vi "2-Rotina de processamento dos dados de caracterização.vi"() -> ()   [LabVIEW 2011]
uses:
  <vilib>/Analysis/NI_AALBase.lvlib
  <vilib>/Analysis/baseanly.llb/Mean (DBL).vi
  <vilib>/Analysis/Matrix/Datatypes/RealMatrix.ctl
  <vilib>/Analysis/Matrix/NI_Matrix.lvlib
  <vilib>/Analysis/NI_AALPro.lvlib
  <vilib>/Analysis/polynomials.llb/1D Polynomial Evaluation (DBL).vi
panel:
  in  "Quantidade \nde Ciclos":dbl
  in  "Massas-padrão\nutilizadas (kg)":dbl[](array[numeric])
  out "Mensagem":string
  out "Regressão Linear:":string
  out "Coeficiente de Determinação:":dbl
  out "Tensão e \nForça do Sinal":cluster{"Y":dbl[], "Y":dbl[]}[](graph)
  # "*1"
  # "*x"
  # "*(x^2)"
  # "*(x^3)"
  # "ROTINA DE PROCESSAMENTO DOS DADOS DE CARACTERIZAÇÃO"
  # "(Um ciclo\ncorresponde\na um \ncarreganento\nseguido de um \ndescarregamento)"
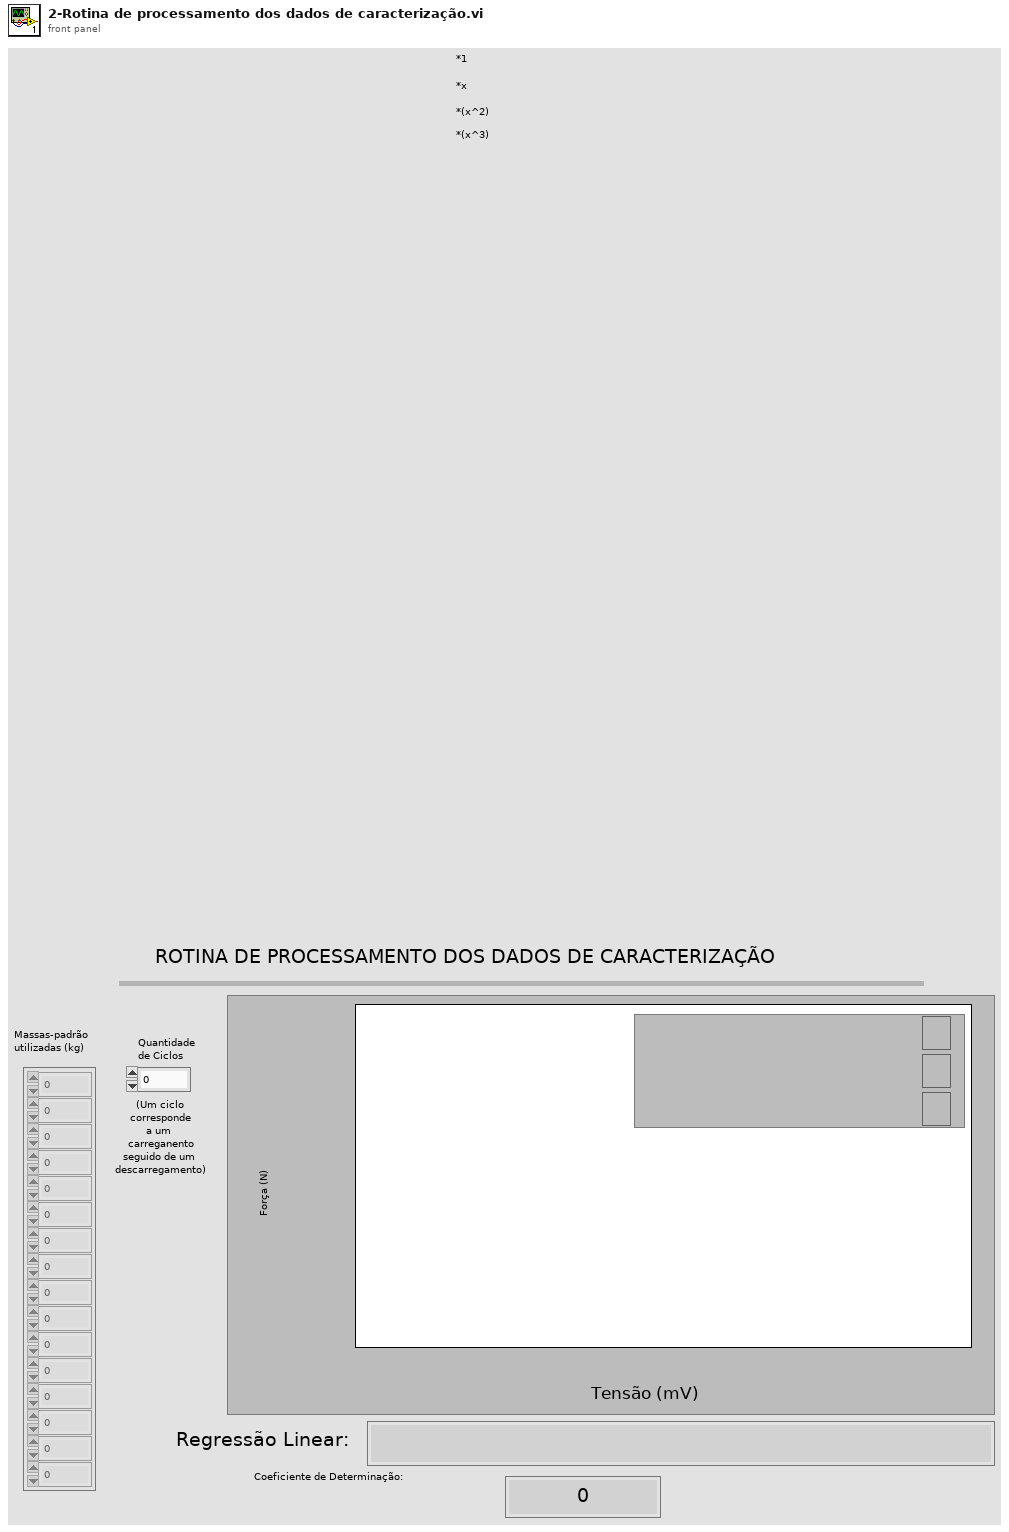
[diagram p1: front panel]
types:
  T1 = typedef "NI_Matrix.lvlib/RealMatrix.ctl" = dbl[][]
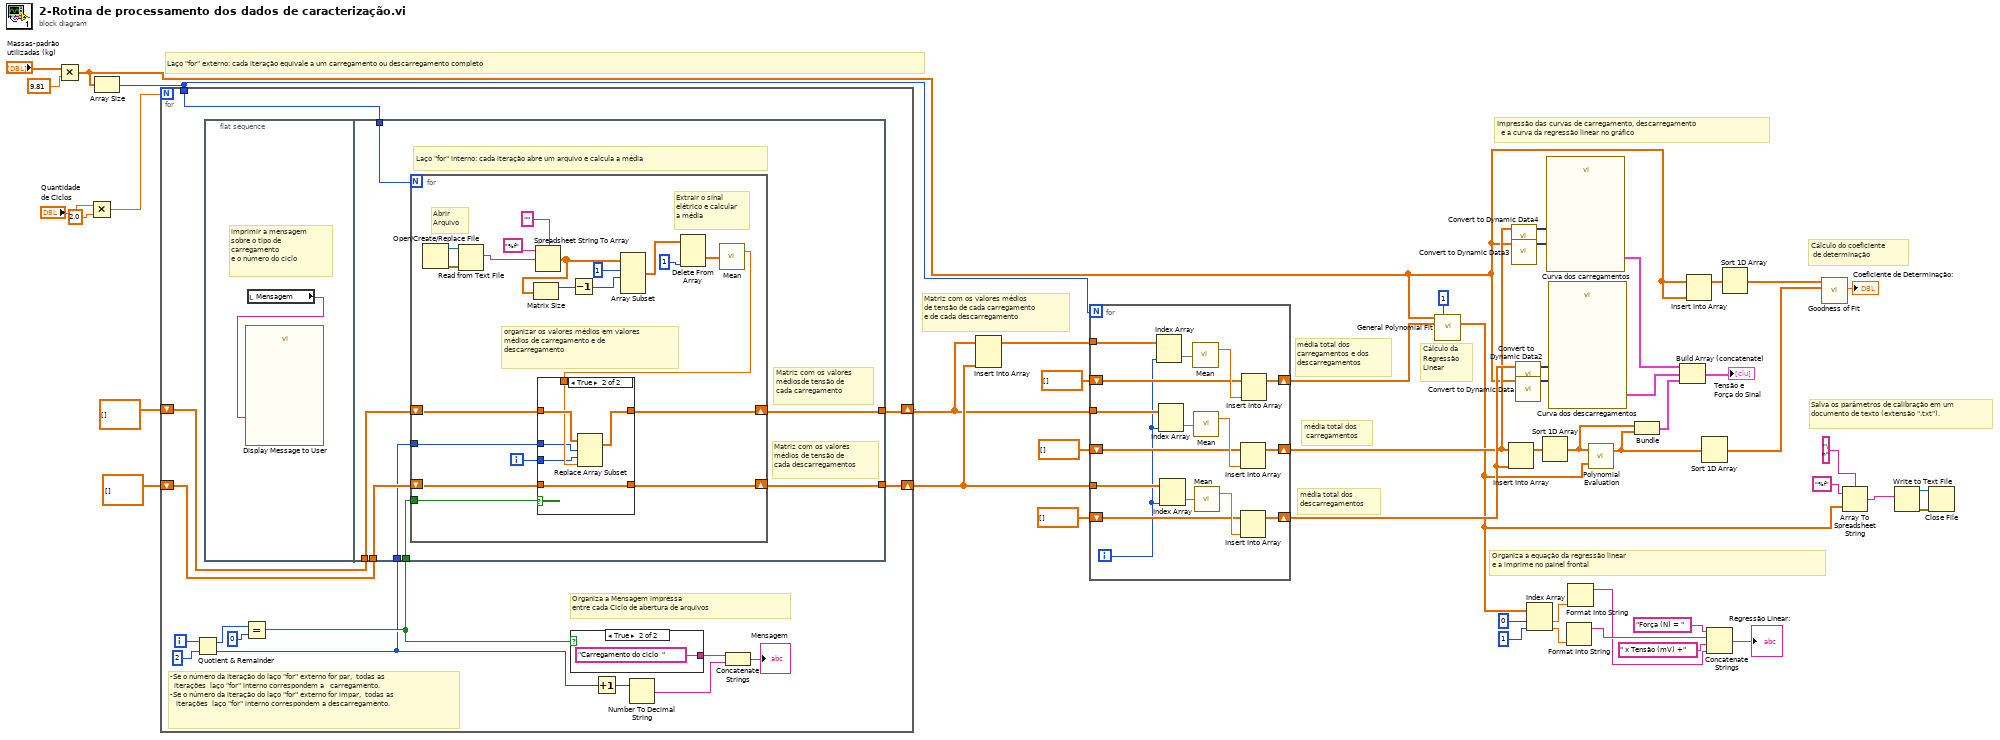
[diagram p0: block diagram]
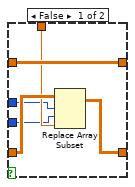
[diagram p2: hidden frame]
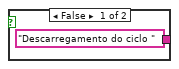
[diagram p3: hidden frame]
diagram:
  # "Salva os parâmetros de calibração em um documento de texto (extensão \".txt\")."
  # "Cálculo do coeficiente\n de determinação"
  # "Impressão das curvas de carregamento, descarregamento\n  e a curva da regressão linear no gráfico"
  # "Cálculo da \nRegressão \nLinear"
  # "Organiza a equação da regressão linear \ne a imprime no painel frontal"
  # "média total dos\ndescarregamentos"
  # "média total dos\n carregamentos"
  # "média total dos \ncarregamentos e dos \ndescarregamentos"
  # "Matriz com os valores médios\nde tensão de cada carregamento \ne de cada descarregamento"
  # "Laço \"for\" externo: cada iteração equivale a um carregamento ou descarregamento completo"
  n1 = Multiply(x="Massas-padrão\nutilizadas (kg)", y=9.81) -> (x*y=w7:dbl[])
  n2 = Multiply(x="Quantidade \nde Ciclos", y=2.0) -> (x*y=w49:dbl)
  n3 = Array Size(array=w7) -> (size(s)=w12:i32)
  n4 = for {
    N: w49 -> [_]
    shift-right: [w57] -> w13
    shift-left: T1 [] ("matrix") -> [w55]
    shift-right: [w56] -> w14
    shift-left: T1 [] ("matrix") -> [w54]
    tunnel: w12 -> [w50]
    i -> [w61]
    # "Organiza a Mensagem impressa\nentre cada Ciclo de abertura de arquivos"
    # "-Se o número da iteração do laço \"for\" externo for par,  todas as  \n  iterações  laço \"for\" interno correspondem a   carregamento.\n-Se o número da iteração do laço \"for\" externo for impar,  todas as\n   iterações  laço \"for\" interno correspondem a descarregamento."
    n5 = Quotient & Remainder(x=w61, y=2) -> (x-y*floor(x/y)=w63:i32, floor(x/y)=w51:i32)
    n6 = flat-sequence {
      tunnel: w50 -> [w72]
      tunnel: w55 -> [w67]
      tunnel: w54 -> [w68]
      tunnel: w52 -> [w71]
      tunnel: w51 -> [w66]
      tunnel: [w70] -> w57
      tunnel: [w69] -> w56
      frame #0 {
        # "imprimir a mensagem\nsobre o tipo de carregamento\ne o número do ciclo"
        n7 = local read "Mensagem"() -> (w65:string)
        n8 = call "Display Message to User"("Message"=w65) -> ()  [unwired: 9 in, 2 out]
      }
      frame #1 {
        # "Laço \"for\" interno: cada iteração abre um arquivo e calcula a média"
        # "Matriz com os valores \nmédios de tensão de \ncada descarregamentos"
        # "Matriz com os valores \nmédiosde tensão de \ncada carregamento"
        n9 = for {
          N: w72 -> [_]
          shift-right: [w78] -> w70
          shift-left: w67 -> [w76]
          shift-right: [w77] -> w69
          shift-left: w68 -> [w79]
          tunnel: w71 -> [w73]
          tunnel: w66 -> [w75]
          i -> [w74]
          # "organizar os valores médios em valores\nmédios de carregamento e de descarregamento"
          # "Abrir \nArquivo"
          # "Extrair o sinal elétrico e calcular a média"
          n10 = Open/Create/Replace File() -> (refnum out=w92:refnum<file>, error out=w90:errorcluster)  [unwired: 6 in, 1 out]
          n11 = Read from Text File(file (use dialog)=w92, error in=w90) -> (text=w89:string)  [unwired: 2 in, 3 out]
          n12 = Spreadsheet String To Array(delimiter (Tab)="", format string="%f", spreadsheet string=w89) -> (array=w83:dbl[][])  [unwired: 1 in]
          n13 = Matrix Size(0:w83) -> (1:w85:i32)  [unwired: 1 out]
          n14 = Decrement(x=w85) -> (x-1=w84:i32)
          n15 = Array Subset(array=w83, index (row)=1 ("row 1"), length (row)=w84) -> (w86:dbl[][])  [unwired: 2 in]
          n16 = Delete From Array(array=w86, index (col)=1 ("disabled index (col)")) -> (deleted portion=w81:dbl[])  [unwired: 2 in, 1 out]
          n17 = call-poly <vilib>:"Mean.vi"("X"=w81) -> ("mean"=w80:dbl)  [unwired: 1 out]
          n18 = case shown="True" w73 {
            tunnel: w80 -> [w95 w101]
            tunnel: w79 -> [w97 w103]
            tunnel: [w96 w104] -> w78
            tunnel: [w98 w103] -> w77
            tunnel: w76 -> [w96 w102]
            tunnel: w75 -> [w94 w99]
            tunnel: w74 -> [w93 w100]
            frame False {
              n19 = Replace Array Subset(array=w97, new element=w95, index (row)=w94, index (col)=w93) -> (w98:T1)
            }
            frame True {
              n20 = Replace Array Subset(array=w102, new element=w101, index (row)=w99, index (col)=w100) -> (w104:T1)
            }
          }
        }
      }
    }
    n21 = Equal?(x=w63, y=0) -> (x = y?=w52:bool)
    n22 = case shown="True" w52 {
      tunnel: ["Descarregamento do ciclo " "Carregamento do ciclo  "] -> w60
      frame False {
      }
      frame True {
      }
    }
    n23 = Increment(x=w51) -> (x+1=w58:i32)
    n24 = Number To Decimal String(number=w58) -> (decimal integer string=w59:string)  [unwired: 1 in]
    n25 = Concatenate Strings(w60, w59) -> (→"Mensagem":string)
  }
  n26 = Insert Into Array(array=w13, new element=w14) -> (w42:T1)  [unwired: 2 in]
  n27 = for {
    N: w12 -> [_]
    tunnel: w13 -> [w122]
    shift-right: [w119] -> w8
    shift-left: dbl[] [] -> [w118]
    shift-right: [w115] -> w9
    shift-left: dbl[] [] -> [w114]
    tunnel: w14 -> [w113]
    tunnel: w42 -> [w111]
    shift-right: [w109] -> w40
    shift-left: dbl[] [] -> [w108]
    i -> [w107]
    n28 = Index Array(array=w111, index (col)=w107) -> (element=w112:dbl[])  [unwired: 1 in]
    n29 = Index Array(array=w122, index (col)=w107) -> (element=w121:dbl[])  [unwired: 1 in]
    n30 = Index Array(array=w113, index (col)=w107) -> (element=w117:dbl[])  [unwired: 1 in]
    n31 = call-poly <vilib>:"Mean.vi"("X"=w112) -> ("mean"=w110:dbl)  [unwired: 1 out]
    n32 = call-poly <vilib>:"Mean.vi"("X"=w121) -> ("mean"=w120:dbl)  [unwired: 1 out]
    n33 = call-poly <vilib>:"Mean.vi"("X"=w117) -> ("mean"=w116:dbl)  [unwired: 1 out]
    n34 = Insert Into Array(array=w118, new element=w120) -> (w119:dbl[])  [unwired: 1 in]
    n35 = Insert Into Array(array=w114, new element=w116) -> (w115:dbl[])  [unwired: 1 in]
    n36 = Insert Into Array(array=w108, new element=w110) -> (w109:dbl[])  [unwired: 1 in]
  }
  n37 = call <vilib>:"General Polynomial Fit.vi"("Y"=w7, "polynomial order"=1, "X"=w40) -> ("Polynomial Coefficients"=w1:dbl[])  [unwired: 9 in, 3 out]
  n38 = Insert Into Array(array=w8, new element=w9) -> (w37:dbl[])  [unwired: 1 in]
  n39 = call "Convert to Dynamic Data4"("Array"=w8) -> ("Dynamic Data Type"=w18:dynamicdata)  [unwired: 3 in]
  n40 = call "Convert to Dynamic Data3"("Array"=w7) -> ("Dynamic Data Type"=w19:dynamicdata)  [unwired: 3 in]
  n41 = call "Convert to Dynamic Data2"("Array"=w9) -> ("Dynamic Data Type"=w38:dynamicdata)  [unwired: 3 in]
  n42 = call "Convert to Dynamic Data"("Array"=w7) -> ("Dynamic Data Type"=w39:dynamicdata)  [unwired: 3 in]
  n43 = Index Array(array=w1, index #1=0 ("index"), index #2=1 ("index")) -> (element #1=w31:dbl, element #2=w30:dbl)
  n44 = Sort 1D Array(array=w37) -> (sorted array=w36:dbl[])
  n45 = call "Curva dos carregamentos"("Y Input"=w19, "X Input"=w18) -> ("XY Graph"=w10:cluster{"Y":dbl[], "Y":dbl[]}[])  [unwired: 3 in, 6 out]
  n46 = call "Curva dos descarregamentos"("Y Input"=w39, "X Input"=w38) -> ("XY Graph"=w11:cluster{"Y":dbl[], "Y":dbl[]}[])  [unwired: 3 in, 6 out]
  n47 = Format Into String(w30) -> (resulting string=w27:string)  [unwired: 3 in, 1 out]
  n48 = Format Into String(w31) -> (resulting string=w26:string)  [unwired: 3 in, 1 out]
  n49 = call-poly <vilib>:"Polynomial Evaluation.vi"("P(x)"=w1, "A"=w36) -> ("P(A)"=w22:dbl[])  [unwired: 1 out]
  n50 = Bundle(w36, "P(A)"=w22) -> (w35:cluster{dbl[], "P(A)":dbl[]})  [unwired: 1 in]
  n51 = Build Array (concatenate)(w10, w11, w35) -> (→"Tensão e \nForça do Sinal":cluster{"Y":dbl[], "P(A)":dbl[]}[])
  n52 = Insert Into Array(array=w7, new element=w7) -> (w24:dbl[])  [unwired: 1 in]
  n53 = Sort 1D Array(array=w22) -> (sorted array=w21:dbl[])
  n54 = Concatenate Strings("Força (N) = ", w27, " x Tensão (mV) +", w26) -> (→"Regressão Linear:":string)
  n55 = Sort 1D Array(array=w24) -> (sorted array=w23:dbl[])
  n56 = call <vilib>:"Goodness of Fit.vi"("Best Fit"=w21, "Y"=w23) -> ("R-square"=→"Coeficiente de Determinação:":dbl)  [unwired: 6 in, 3 out]
  n57 = Array To Spreadsheet String(delimiter (Tab)="\n", array=w1, 3:"%f" ("format string")) -> (spreadsheet string=w2:string)
  n58 = Write to Text File(text=w2) -> (refnum out=w4:refnum<file>, error out=w3:errorcluster)  [unwired: 3 in, 1 out]
  n59 = Close File(refnum=w4, error in=w3) -> ()  [unwired: 2 out]
